vi "Send successful actuator to BMC.vi"(8 "error in (no error)":errorcluster, 9 "actuator in":dbl, 10 "current plus 1 in":dbl[](array[numeric]), 11 "RSA in":refnum<class "RSA.lvclass">) -> (0 "error out":errorcluster, 3 "RSA out":refnum<class "RSA.lvclass">)   [LabVIEW 2012, in "RSA.lvclass"]
uses:
  RSA.lvclass
  <vilib>/Distrio/Murmex/Murmex/Murmex.lvclass
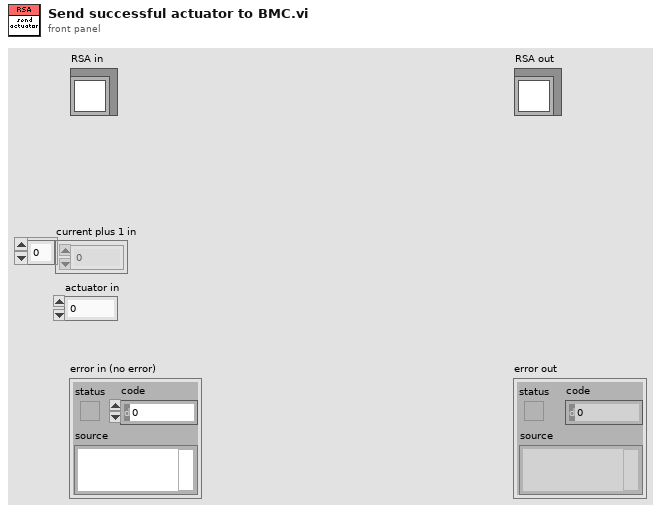
[diagram p1: front panel]
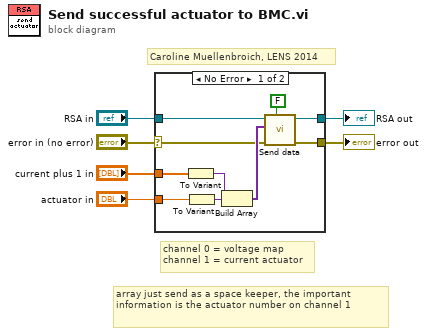
[diagram p0: block diagram]
diagram:
  # "array just send as a space keeper, the important information is the actuator number on channel 1"
  # "channel 0 = voltage map\nchannel 1 = current actuator"
  # "Caroline Muellenbroich, LENS 2014"
  n1 = case shown="No Error" "error in (no error)" {
    selector: "error in (no error)" -> [w10 w18]
    tunnel: [w9 w18] -> w5
    tunnel: [w11 w17] -> w3
    tunnel: "RSA in" -> [w12 w17]
    tunnel: "current plus 1 in" -> [w8 _]
    tunnel: "actuator in" -> [w7 _]
    frame No Error {
      n2 = To Variant(anything=w8) -> (Variant=w16:variant)
      n3 = To Variant(anything=w7) -> (Variant=w15:variant)
      n4 = Build Array(w16, w15) -> (w14:variant[])
      n5 = call <vilib>:"Send data.vi"("is finalised data? (T)"=FALSE, "error in (no error)"=w10, "data (channels array)"=w14, "Murmex in"=w12) -> ("error out"=w9:errorcluster, "Murmex out"=w11:refnum<class "RSA.lvclass">)  [unwired: 6 in]
    }
    frame Error {
    }
  }
  "error out" <- w5
  "RSA out" <- w3
